vi "test control.vi"() -> ()   [LabVIEW 2017, in "Signal Selector.lvlib"]
uses:
  Selection Folder/Selection.xctl
  Selection Folder/Signal types.ctl
  Signal Selector.lvlib
panel:
  in  "stop":bool
  out "Index(es)":i32[][](array[numeric])
  out "Array":T1[](array[typedef])
  in  "Selection":cluster{"Type":T1, "Index(es)":i32[]}[](xcontrol)
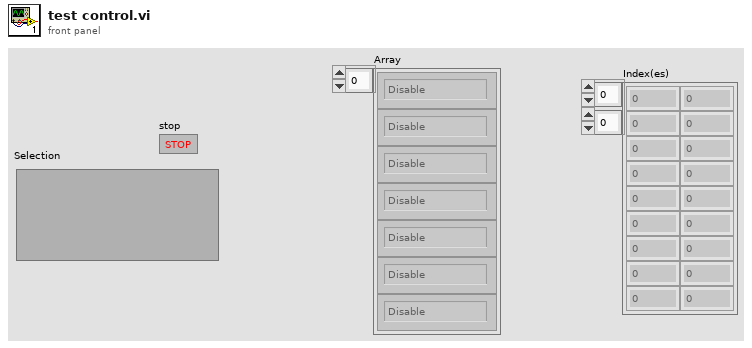
[diagram p1: front panel]
types:
  T1 = typedef "Selection.xctl/Signal types.ctl" = enum16{"Disable", "Frequency", "Phasor Mag", "Phasor Ang", "Angle Diff"}
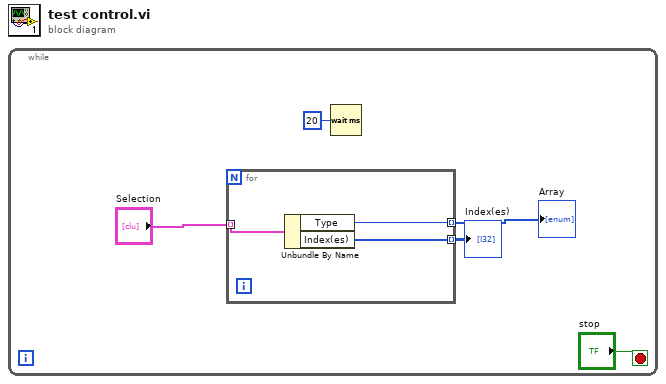
[diagram p0: block diagram]
diagram:
  n1 = while {
    stop <- "stop" stop-if-true
    n2 = for {
      tunnel: "Selection" -> [w8] mode=indexing
      tunnel: [w7] -> w4 mode=indexing
      tunnel: [w6] -> w3 mode=indexing
      n3 = Unbundle By Name(w8) -> ("Type"=w7:T1, "Index(es)"=w6:i32[])
    }
    "Array" <- w4
    "Index(es)" <- w3
    n4 = Wait (ms)(milliseconds to wait=u32 20) -> ()  [unwired: 1 out]
  }
